vi "GetQualifiedName.vi"(8 "error in (no error)":errorcluster, 11 "Module ID":i32=-1) -> (0 "error out":errorcluster, 1 "timed out?":bool, 2 "Reply Payload":T1)   [LabVIEW 2014, in "Configurable.lvlib"]
doc: "Requests the module's Fully Qualified Name\n_____\nCreated using Delacor QMH Event Scripter 4.0.0.68."
uses:
  Configurable.lvlib
  GetQualifiedName (Reply Payload)--cluster.ctl
  GetQualifiedName Argument--cluster.ctl
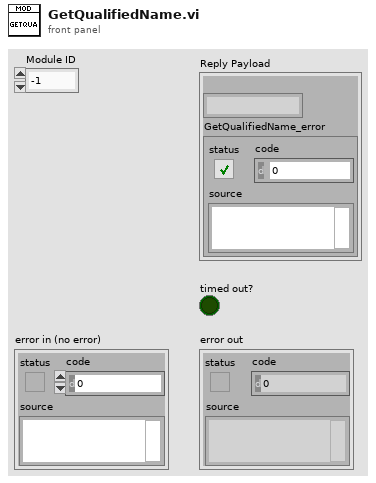
[diagram p1: front panel]
types:
  T1 = typedef "Configurable.lvlib/GetQualifiedName (Reply Payload)--cluster.ctl" = cluster{"Fully Qualified Name":string, "GetQualifiedName_error":errorcluster}
  T2 = typedef "Configurable.lvlib/GetQualifiedName Argument--cluster.ctl" = cluster{"Module ID":i32, "Fully Qualified Name":string, "Wait Notifier":refnum<notifier>}
  T3 = typedef "Configurable.lvlib/Request Events--cluster.ctl" = cluster{"Stop Module":refnum<user-event>, "Show Panel":refnum<user-event>, "Hide Panel":refnum<user-event>, "Show Diagram":refnum<user-event>, "Get Module Execution Status":refnum<user-event>, "GetQualifiedName":refnum<user-event>}
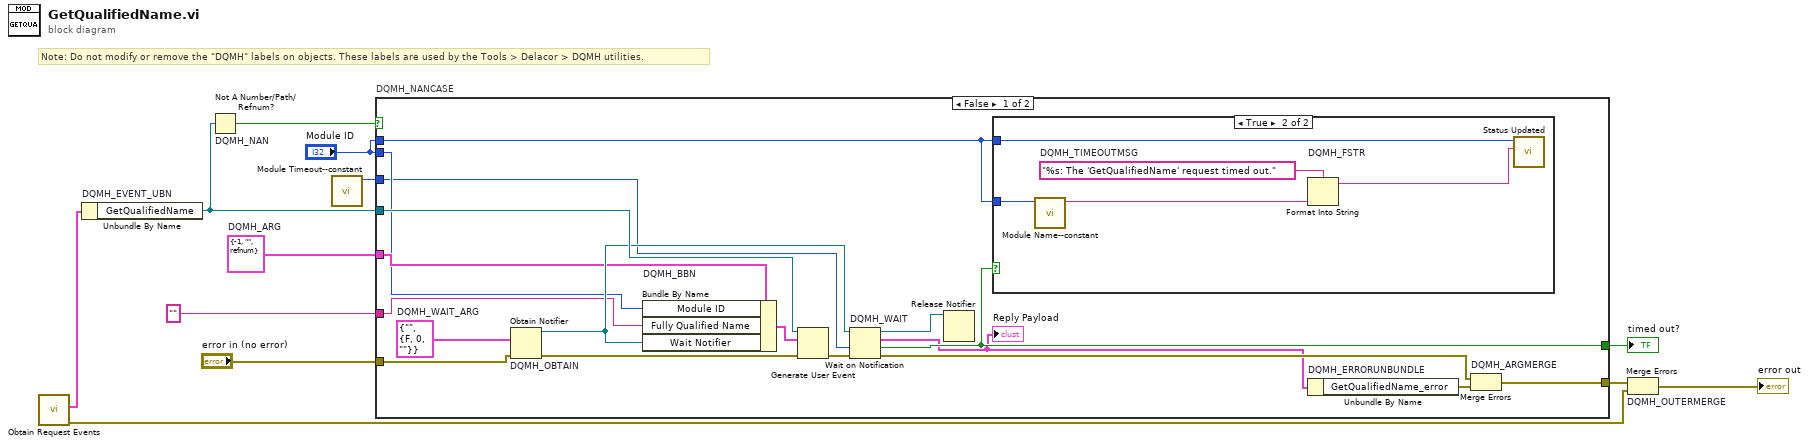
[diagram p0: block diagram]
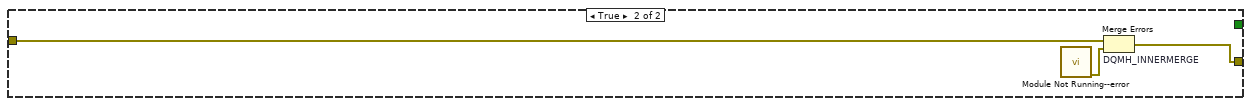
[diagram p3: hidden frame]
diagram:
  w6 = T2 {"Module ID"=-1, "Fully Qualified Name"="", "Wait Notifier"=refnum}  # DQMH_ARG
  # "Note: Do not modify or remove the \"DQMH\" labels on objects. These labels are used by the Tools > Delacor > DQMH utilities."
  n1 = call "Obtain Request Events.vi"() -> ("error out"=w2:errorcluster, "Configurable Request Events"=w1:T3)  [unwired: 10 in]
  n2 = Unbundle By Name "DQMH_EVENT_UBN"(w1) -> ("GetQualifiedName"=w10:refnum<user-event>)
  n3 = Not A Number/Path/Refnum? "DQMH_NAN"(number/path/refnum=w10) -> (NaN/Path/Refnum?=w9:bool)
  n4 = call "Module Timeout--constant.vi"() -> ("Module Timeout"=w4:i32)  [unwired: 11 in]
  n5 = case "DQMH_NANCASE" shown="False" w9 {
    tunnel: "error in (no error)" -> [w30 w38]
    tunnel: w10 -> [w28 _]
    tunnel: [w21 w37] -> w7
    tunnel: [w22 _] -> w8
    tunnel: w6 -> [w17 _]
    tunnel: "Module ID" -> [w16 _]
    tunnel: "" ("Fully Qualified Name") -> [w15 _]
    tunnel: w4 -> [w14 _]
    tunnel: "Module ID" -> [w13 _]
    frame False {
      w26 = T1 {"Fully Qualified Name"="", "GetQualifiedName_error"={"status"=FALSE, "code"=0, "source"=""}}  # DQMH_WAIT_ARG
      n6 = Obtain Notifier "DQMH_OBTAIN"(notification data type=w26, error in (no error)=w30) -> (notifier out=w24:refnum<notifier>, error out=w27:errorcluster)  [unwired: 2 in, 1 out]
      n7 = Bundle By Name "DQMH_BBN"(cluster=w17, "Module ID"=w16, "Fully Qualified Name"=w15, "Wait Notifier"=w24) -> (w18:T2)
      n8 = Generate User Event(user event=w28, event data cluster=w18, error in=w27) -> (error out=w29:errorcluster)  [unwired: 1 in, 1 out]
      n9 = Wait on Notification "DQMH_WAIT"(notifier=w24, timeout in ms (-1)=w14, error in (no error)=w29) -> (notifier out=w23:refnum<notifier>, notification=w19:T1, timed out?=w22:bool, error out=w25:errorcluster)  [unwired: 1 in]
      "Reply Payload" <- w19
      n10 = Release Notifier(notifier=w23) -> ()  [unwired: 2 in, 3 out]
      n11 = case shown="True" w22 {
        tunnel: w13 -> [_ w32]
        tunnel: w13 -> [_ w31]
        frame False {
        }
        frame True {
          w35 = "%s: The 'GetQualifiedName' request timed out."  # DQMH_TIMEOUTMSG
          n12 = call "Module Name--constant.vi"("Module ID"=w31) -> ("Module Name"=w34:string)  [unwired: 10 in]
          n13 = Format Into String "DQMH_FSTR"(format string=w35, w34) -> (resulting string=w33:string)  [unwired: 2 in, 1 out]
          n14 = call "Status Updated.vi"("Status"=w33, "Module ID"=w32) -> ()  [unwired: 9 in, 1 out]
        }
      }
      n15 = Unbundle By Name "DQMH_ERRORUNBUNDLE"(w19) -> ("GetQualifiedName_error"=w20:errorcluster)
      n16 = Merge Errors "DQMH_ARGMERGE"(w25, w20) -> (w21:errorcluster)
    }
    frame True {
      n17 = call "Module Not Running--error.vi"() -> ("error out"=w36:errorcluster)  [unwired: 11 in]
      n18 = Merge Errors "DQMH_INNERMERGE"(w38, w36) -> (w37:errorcluster)
    }
  }
  "timed out?" <- w8
  n19 = Merge Errors "DQMH_OUTERMERGE"(w7, w2) -> (→"error out":errorcluster)
